vi "VariableGroup.vi"(10 "DisplayList":string[](array[string]), 11 "GroupName":string) -> (3 "VariableGroup":refnum<class "VariableGroup.lvclass">)   [LabVIEW 2013, in "VariableManagerAPI.lvlib"]
doc: "Return Variable group object.\nThe object contains given values (optional).\nData can be accessed through property node.\n\n<B>GroupName</B>: the name of the group\n<B>DisplayList</B>: the list of variable names that are in the group."
uses:
  VariableManagerAPI.lvlib
  VariableGroup/VariableGroup.lvclass
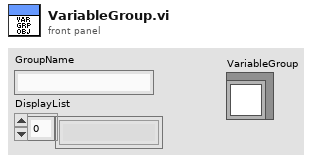
[diagram p1: front panel]
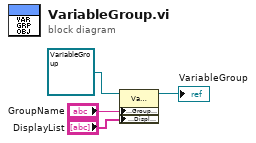
[diagram p0: block diagram]
diagram:
  n1 = property class="VariableGroup.lvclass"(reference=refnum<class "VariableGroup.lvclass"> refnum ("VariableGroup.lvclass"), "Accessors:GroupName"="GroupName", "Accessors:DisplayList"="DisplayList") -> (reference out=→"VariableGroup":refnum<class "VariableGroup.lvclass">)  [unwired: 1 in, 1 out]
